vi "Magnet Limits.vi"(0 "instrument.PPMS1":refnum<class "instrument.PPMS1.lvclass">, 5 "Helium (%)":dbl, 7 "Target Field (Oe)":dbl, 9 "Mode":T1, 11 "error in (no error)":errorcluster) -> (4 "instrument.PPMS1 out":refnum<class "instrument.PPMS1.lvclass">, 8 "Limited Field (Oe)":dbl, 10 "Mode out":T1, 15 "error out":errorcluster)   [LabVIEW 2016, in "instrument.PPMS1.lvclass"]
uses:
  instrument.PPMS1.lvclass
  <userlib>/LevyLab/Levylab Instruments/Instrument Types/Cryostat/Typedefs/Magnet Mode--Enum.ctl
  <userlib>/LevyLab/Levylab Instruments/Instrument Types/Cryostat/Instrument.Cryostat.lvclass
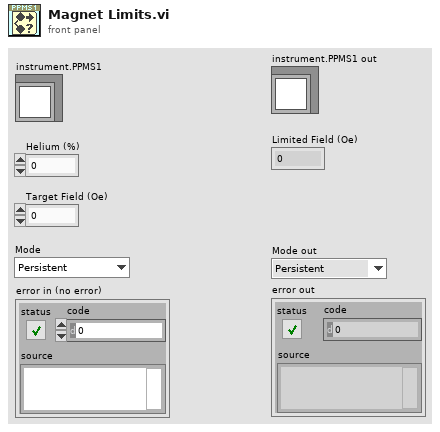
[diagram p1: front panel]
types:
  T1 = typedef "Instrument.Cryostat.lvclass/Magnet Mode--Enum.ctl" = enum16{"Persistent", "Driven"}
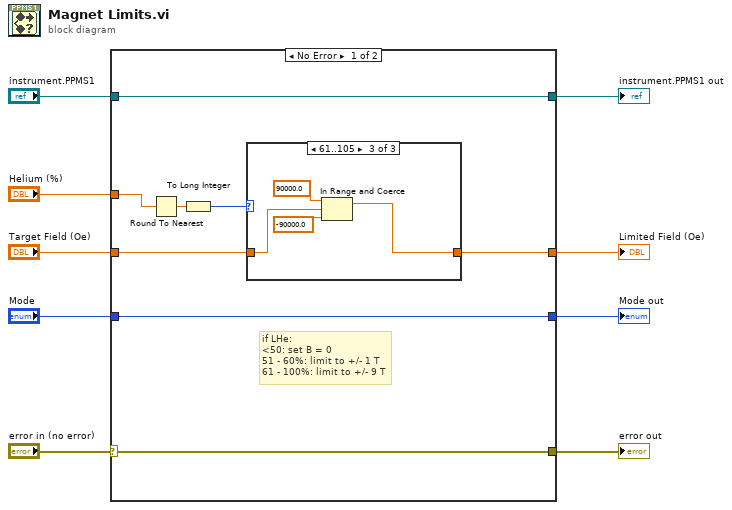
[diagram p0: block diagram]
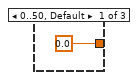
[diagram p2: hidden frame]
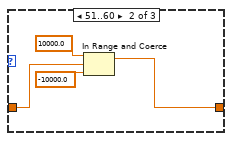
[diagram p3: hidden frame]
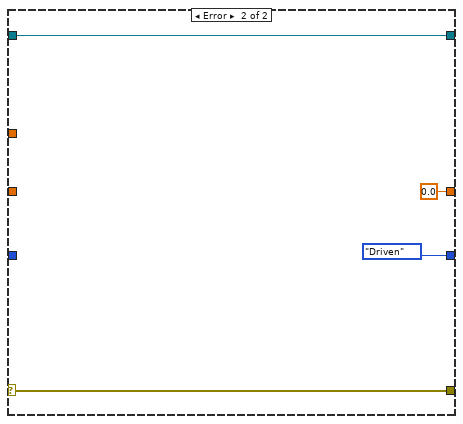
[diagram p4: hidden frame]
diagram:
  n1 = case shown="No Error" "error in (no error)" {
    selector: "error in (no error)" -> [w16 w30]
    tunnel: "Target Field (Oe)" -> [w12 _]
    tunnel: [w11 0.0 ("upper limit")] -> w7
    tunnel: "instrument.PPMS1" -> [w17 w29]
    tunnel: [w17 w29] -> w8
    tunnel: [w16 w30] -> w3
    tunnel: [w10 Magnet_Mode--Enum."Driven" ("Mode")] -> w2
    tunnel: "Mode" -> [w10 _]
    tunnel: "Helium (%)" -> [w13 _]
    frame No Error {
      # "if LHe:\n<50: set B = 0\n51 - 60%: limit to +/- 1 T\n61 - 100%: limit to +/- 9 T"
      n2 = Round To Nearest(number=w13) -> (nearest integer value=w15:dbl)
      n3 = To Long Integer(number=w15) -> (32bit integer=w14:i32)
      n4 = case shown="61..105" w14 {
        tunnel: w12 -> [_ w22 w26]
        tunnel: [0.0 ("upper limit") w19 w23] -> w11
        frame 0..50, Default {
        }
        frame 51..60 {
          n5 = In Range and Coerce(upper limit=10000.0, x=w22, lower limit=-10000.0) -> (coerced(x)=w19:dbl)  [unwired: 1 out]
        }
        frame 61..105 {
          n6 = In Range and Coerce(upper limit=90000.0, x=w26, lower limit=-90000.0) -> (coerced(x)=w23:dbl)  [unwired: 1 out]
        }
      }
    }
    frame Error {
    }
  }
  "Limited Field (Oe)" <- w7
  "instrument.PPMS1 out" <- w8
  "Mode out" <- w2
  "error out" <- w3
